vi "get crate offset.vi"(8 "error in":errorcluster, 11 "Crate":i32) -> (0 "error out":errorcluster, 3 "Start offset":i32)   [LabVIEW 2018]
uses:
  CAEN globals.vi
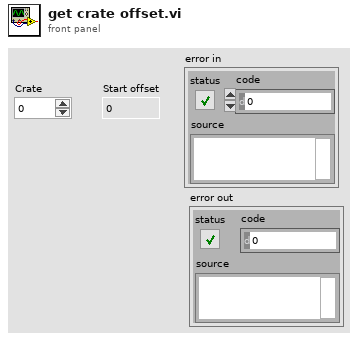
[diagram p1: front panel]
types:
  T1 = typedef "crate.ctl" = cluster{"CAENet Address":i32, "Crate Model":string, "Firmware Version":string, "Crate Map":T2[], "Total Channels":i32}
  T2 = typedef "card.ctl" = cluster{"Slot Number":i32, "Card Model":string, "Num Channels":i32, "Polarity":string, "Vmax":dbl, "Imax":dbl, "Revision":string}
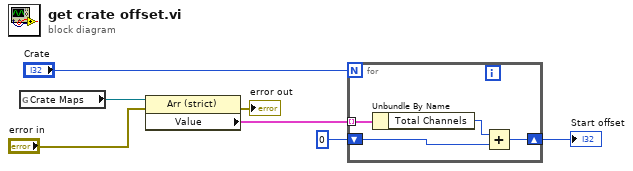
[diagram p0: block diagram]
diagram:
  n1 = global read "CAEN globals.vi" "Crate Maps"() -> (w3:refnum<vi>)
  n2 = property class="Arr (strict)"(reference=w3, error in="error in") -> (error out=→"error out":errorcluster, "Value"=w5:T1[])  [unwired: 1 out]
  n3 = for {
    N: "Crate" -> [_]
    tunnel: w5 -> [w11] mode=indexing
    shift-right: [w9] -> w7
    shift-left: 0 ("Total Channels") -> [w8]
    n4 = Unbundle By Name(w11) -> ("Total Channels"=w10:i32)
    n5 = Add(x=w10, y=w8) -> (x+y=w9:i32)
  }
  "Start offset" <- w7
